vi "Read Sampling Rate.vi"(8 "error in (no error)":errorcluster, 11 "LINX-ADS1X15 in":refnum<class "LINX-ADS1256.lvclass">) -> (0 "error out":errorcluster, 2 "Sampling Rate":T1, 3 "LINX-ADS1X15 out":refnum<class "LINX-ADS1256.lvclass">)   [LabVIEW 2020, in "LINX-ADS1256.lvclass"]
uses:
  LINX-ADS1256.lvclass
  LINX-ADS1256.lvclass/LINX-ADS1256.ctl
  Sample Rate.ctl
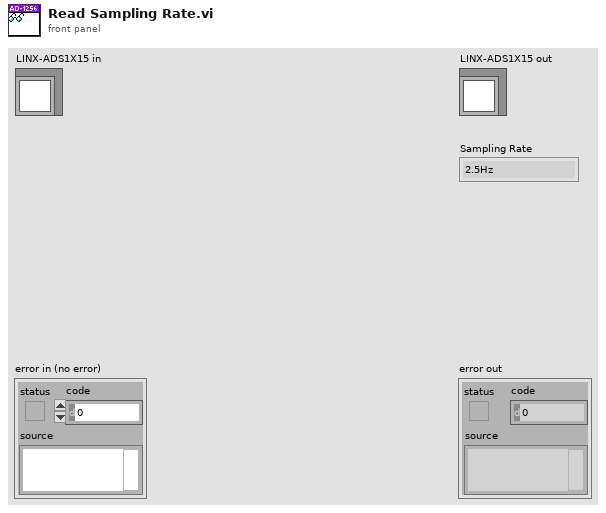
[diagram p1: front panel]
types:
  T1 = typedef "LINX-ADS1256.lvclass/Sample Rate.ctl" = enum16{"2.5Hz", "5Hz", "10Hz", "15Hz", "25Hz", "30Hz", "50Hz", "60Hz", "100Hz", "500Hz", "1000Hz", "2000Hz", "3750Hz", "7500Hz", "15000Hz", "30000Hz"}
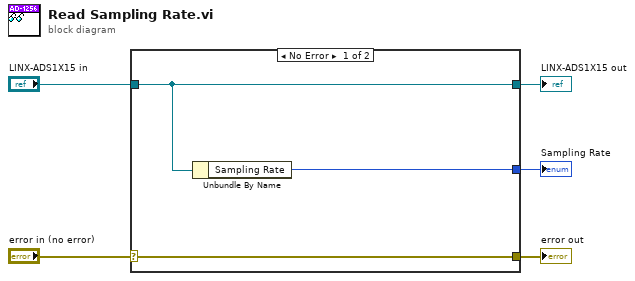
[diagram p0: block diagram]
diagram:
  n1 = case shown="No Error" "error in (no error)" {
    selector: "error in (no error)" -> [w8 w9]
    tunnel: [w8 w9] -> w4
    tunnel: [w7 w10] -> w2
    tunnel: "LINX-ADS1X15 in" -> [w7 w10]
    tunnel: [w6 _] -> w1
    frame No Error {
      n2 = Unbundle By Name(w7) -> ("Sampling Rate"=w6:T1)
    }
    frame Error {
    }
  }
  "error out" <- w4
  "LINX-ADS1X15 out" <- w2
  "Sampling Rate" <- w1
